vi "Command Read.vi"(7 "Error In":errorcluster, 9 "DebugCommandRead?":bool) -> (0 "Error Out":errorcluster, 1 "value 2":dbl[](array[numeric]), 2 "value":dbl[](array[numeric]), 3 "command":string[](array[string]))   [LabVIEW 2017]
uses:
  <vilib>/Rock Robotics/WPI/DriverStation/WPI_DriverStationPositionInfo.ctl
  <vilib>/Utility/file.llb/Read Delimited Spreadsheet (string).vi
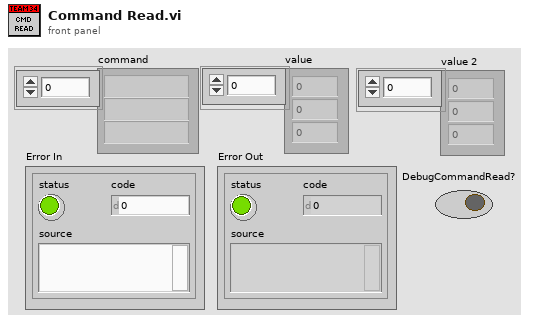
[diagram p1: front panel]
types:
  T1 = typedef "WPI_DriverStationPositionInfo.ctl" = enum16{"1", "2", "3"}
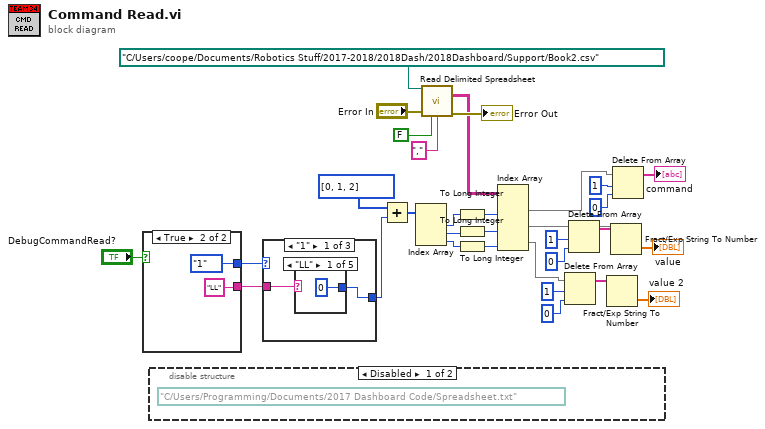
[diagram p0: block diagram]
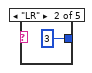
[diagram p2: hidden frame]
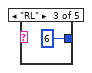
[diagram p3: hidden frame]
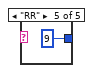
[diagram p5: hidden frame]
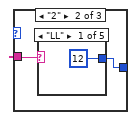
[diagram p6: hidden frame]
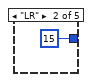
[diagram p7: hidden frame]
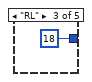
[diagram p8: hidden frame]
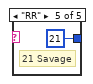
[diagram p10: hidden frame]
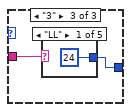
[diagram p11: hidden frame]
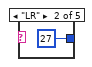
[diagram p12: hidden frame]
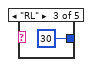
[diagram p13: hidden frame]
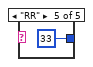
[diagram p15: hidden frame]
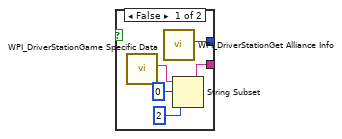
[diagram p16: hidden frame]
diagram:
  n1 = case shown="True" "DebugCommandRead?" {
    tunnel: [w34 WPI_DriverStationPositionInfo."1" ("Position")] -> w26
    tunnel: [w33 "LL" ("Game Specific Data")] -> w25
    frame False {
      n2 = call <vilib>:"WPI_DriverStationGame Specific Data.vi"() -> ("Game Specific Data"=w37:string)  [unwired: 11 in]
      n3 = call <vilib>:"WPI_DriverStationGet Alliance Info.vi"() -> ("Position"=w34:T1)  [unwired: 6 in, 5 out]
      n4 = String Subset(string=w37, offset (0)=0, length (rest)=2 ("length (rest)")) -> (substring=w33:string)
    }
    frame True {
    }
  }
  n5 = disable-structure shown="Disabled" {
    frame Disabled {
      (unwired) path "C:/Users/Programming/Documents/2017 Dashboard Code/Spreadsheet.txt" ("file path (dialog if empty)")
    }
    frame Enabled {
    }
  }
  n6 = case shown="\"1\"" w26 {
    tunnel: w25 -> [w41 w47 w52]
    tunnel: [w40 w46 w53] -> w24
    frame "1" {
      n7 = case shown="\"LL\"" w41 {
        tunnel: [u64 0 u64 3 u64 6 _ u64 9] -> w40
        frame "LL" {
        }
        frame "LR" {
        }
        frame "RL" {
        }
        frame Default {
        }
        frame "RR" {
        }
      }
    }
    frame "2" {
      n8 = case shown="\"LL\"" w47 {
        tunnel: [u64 12 u64 15 u64 18 _ u64 21] -> w46
        frame "LL" {
        }
        frame "LR" {
        }
        frame "RL" {
        }
        frame Default {
        }
        frame "RR" {
          # "21 Savage"
        }
      }
    }
    frame "3" {
      n9 = case shown="\"LL\"" w52 {
        tunnel: [u64 24 u64 27 u64 30 _ u64 33] -> w53
        frame "LL" {
        }
        frame "LR" {
        }
        frame "RL" {
        }
        frame Default {
        }
        frame "RR" {
        }
      }
    }
  }
  n10 = Add(x=u64[] [0, 1, 2] ("Array"), y=w24) -> (x+y=w31:u64[])
  n11 = Index Array(array=w31) -> (element #1=w16:u64, element #2=w19:u64, element #3=w21:u64)  [unwired: 3 in]
  n12 = call-poly <vilib>:"Read Delimited Spreadsheet.vi"("file path (dialog if empty)"=path "C:/Users/coope/Documents/Robotics Stuff/2017-2018/2018Dash/2018Dashboard/Support/Book2.csv", "error in (no error)"="Error In", "transpose? (F)"=FALSE, "delimiter (\\t)"="," ("delimiter (\\t)")) -> ("all rows"=w15:string[][], "error out"=→"Error Out":errorcluster)  [unwired: 6 in, 4 out]
  n13 = To Long Integer(number=w16) -> (32bit integer=w17:i32)
  n14 = To Long Integer(number=w19) -> (32bit integer=w18:i32)
  n15 = To Long Integer(number=w21) -> (32bit integer=w20:i32)
  n16 = Index Array(array=w15, index (col) #1=w17, index (col) #2=w18, index (col) #3=w20) -> (element #1=w12:string[], element #2=w7:string[], element #3=w4:string[])  [unwired: 3 in]
  n17 = Delete From Array(array=w4, length=1, index=0) -> (array with subset deleted=w3:string[])  [unwired: 1 out]
  n18 = Delete From Array(array=w7, length=1, index=0) -> (array with subset deleted=w10:string[])  [unwired: 1 out]
  n19 = Fract/Exp String To Number(string=w3) -> (number=→"value 2":dbl[])  [unwired: 3 in, 1 out]
  n20 = Fract/Exp String To Number(string=w10) -> (number=→"value":dbl[])  [unwired: 3 in, 1 out]
  n21 = Delete From Array(array=w12, length=1, index=0) -> (array with subset deleted=→"command":string[])  [unwired: 1 out]
